vi "GetEnumFeatureEntrys.vi"(8 "pFeatureName":string, 9 "EntryNum":u32, 10 "handle":i64, 11 "error in (no error)":errorcluster) -> (2 "pLbEnumEntryList":string, 3 "error out":errorcluster)   [LabVIEW 2016]
uses:
  MVSDKmd.dll
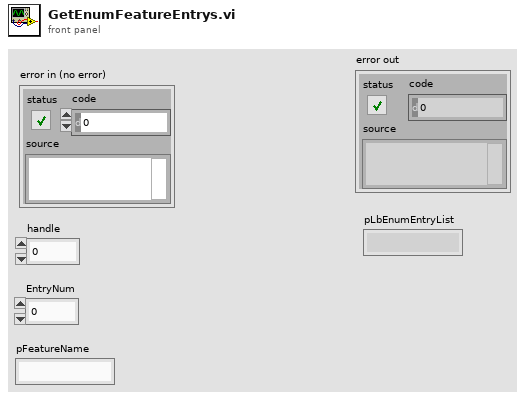
[diagram p1: front panel]
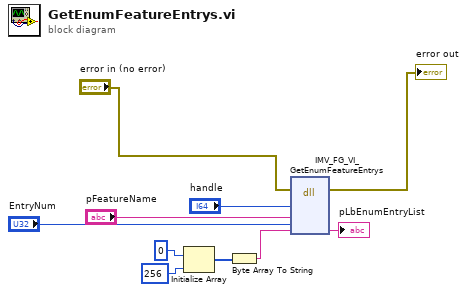
[diagram p0: block diagram]
diagram:
  n1 = Initialize Array(u8 0, 256) -> (w5:u8[])
  n2 = Byte Array To String(unsigned byte array=w5) -> (string=w4:string)
  n3 = dll-call lib="MVSDKmd.dll" fn="IMV_FG_VI_GetEnumFeatureEntrys"(error in="error in (no error)", "handle"="handle", "pFeatureName"="pFeatureName", "EntryNum"="EntryNum", "pLbEnumEntryList"=w4) -> (error out=→"error out":errorcluster, "pLbEnumEntryList"=→"pLbEnumEntryList":string)  [unwired: 6 in, 1 out]
